vi "print.vi"(6 "ShowType?":bool, 8 "error in (no error)":errorcluster, 11 "Expression":T1) -> (0 "error out":errorcluster, 3 "String":string)   [LabVIEW 2020]
uses:
  ExpressionType.ctl
  Expression.ctl
  ClosureData.ctl
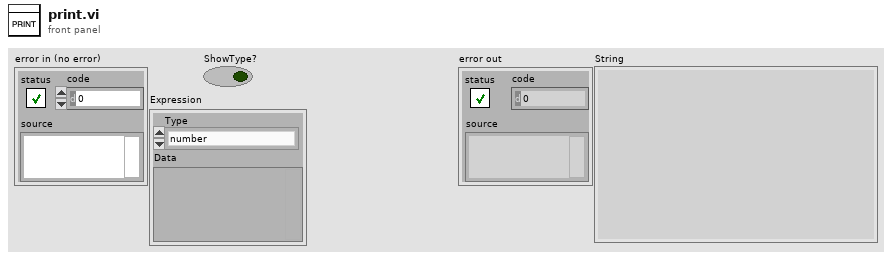
[diagram p1: front panel]
types:
  T1 = typedef "Expression.ctl" = cluster{"Type":T2, "Data":variant}
  T2 = typedef "ExpressionType.ctl" = enum16{"number", "string", "symbol", "primitive", "list", "closure", "macro", "nil", "error"}
  T3 = typedef "ClosureData.ctl" = cluster{"arguments":string[], "code":T1}
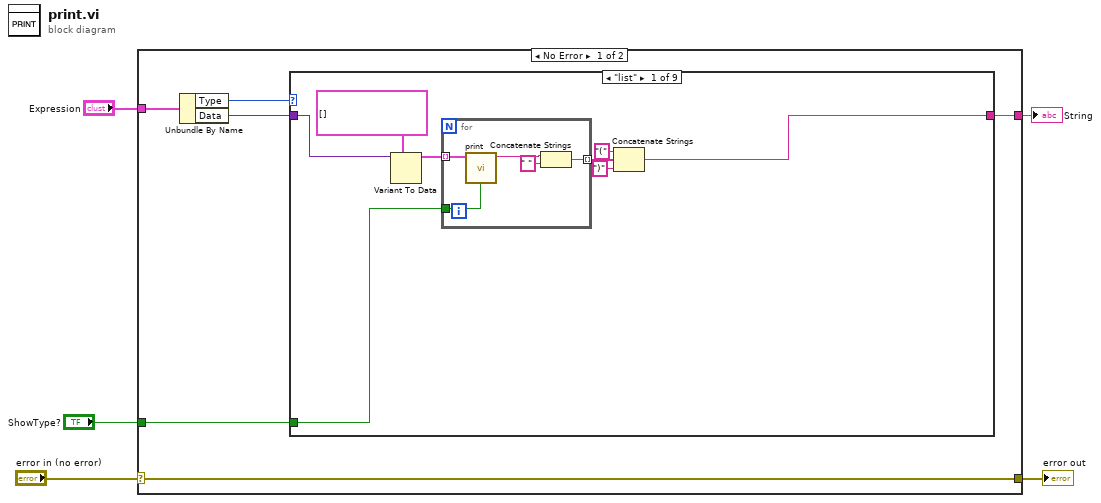
[diagram p0: block diagram]
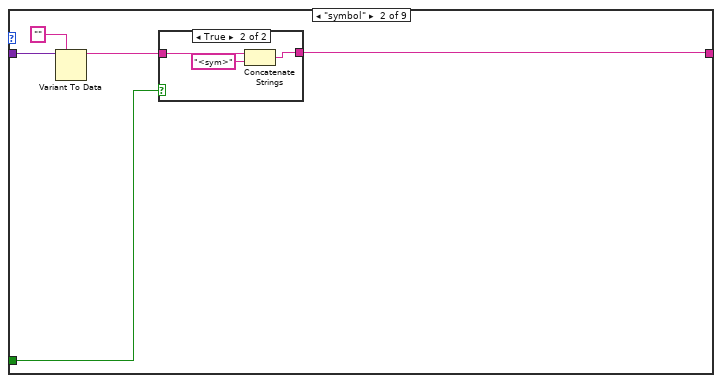
[diagram p2: hidden frame]
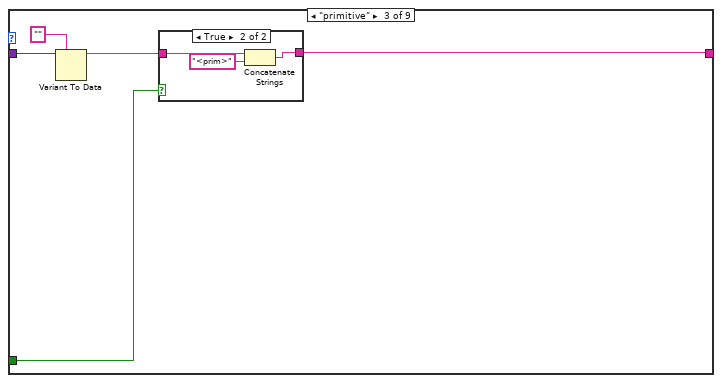
[diagram p4: hidden frame]
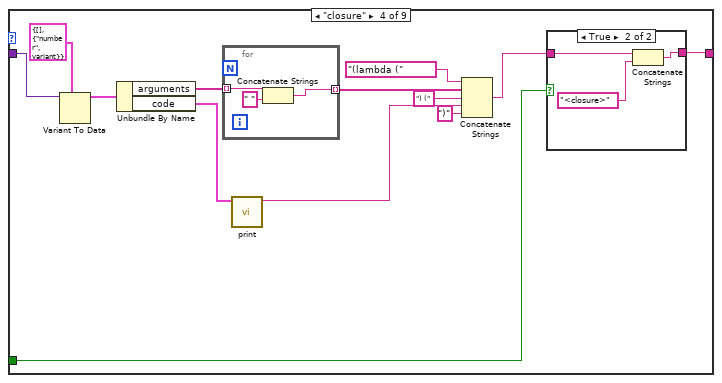
[diagram p6: hidden frame]
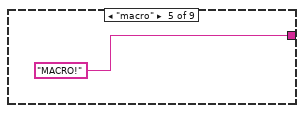
[diagram p8: hidden frame]
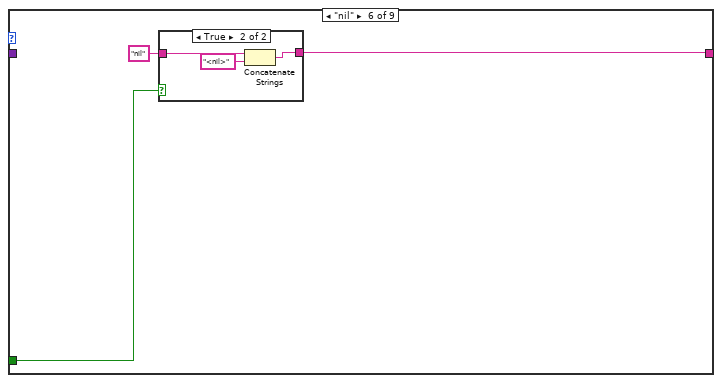
[diagram p9: hidden frame]
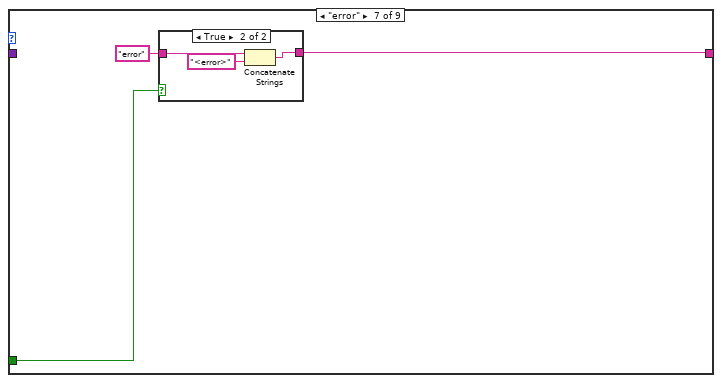
[diagram p11: hidden frame]
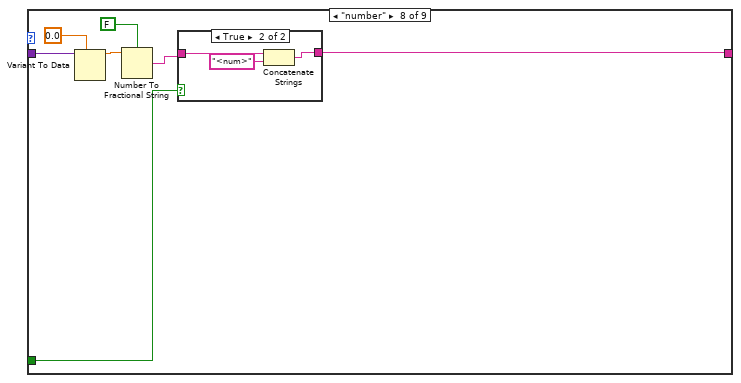
[diagram p13: hidden frame]
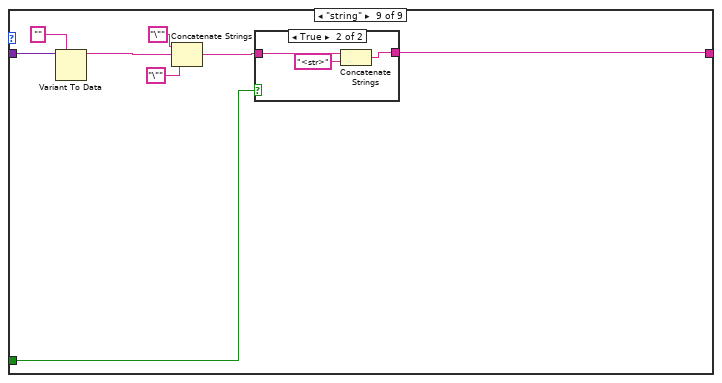
[diagram p15: hidden frame]
diagram:
  n1 = case shown="No Error" "error in (no error)" {
    selector: "error in (no error)" -> [w11 w101]
    tunnel: [w11 w101] -> w4
    tunnel: "Expression" -> [w10 _]
    tunnel: [w7 _] -> w3
    tunnel: "ShowType?" -> [w6 _]
    frame No Error {
      n2 = Unbundle By Name(w10) -> ("Type"=w9:T2, "Data"=w8:variant)
      n3 = case shown="\"list\"" w9 {
        tunnel: w8 -> [w19 w29 w38 w55 _ _ _ w84 w96]
        tunnel: [w14 w26 w35 w54 "MACRO!" w66 w73 w83 w93] -> w7
        tunnel: w6 -> [w13 w25 w34 w53 _ w65 w72 w82 w94]
        frame "list" {
          n4 = Variant To Data(type=T1[] [], Variant=w19) -> (data=w18:T1[])  [unwired: 1 in, 1 out]
          n5 = for {
            tunnel: w18 -> [w22] mode=indexing
            tunnel: [w23] -> w17 mode=indexing
            tunnel: w13 -> [w21]
            n6 = call "print.vi"("ShowType?"=w21, "Expression"=w22) -> ("String"=w20:string)  [unwired: 8 in, 1 out]
            n7 = Concatenate Strings(w20, " " ("string")) -> (w23:string)
          }
          n8 = Concatenate Strings("(" ("string"), w17, ")" ("string")) -> (w14:string)
        }
        frame "symbol" {
          n9 = Variant To Data(type="", Variant=w29) -> (data=w27:string)  [unwired: 1 in, 1 out]
          n10 = case shown="True" w25 {
            tunnel: [w30 w32] -> w26
            tunnel: w27 -> [w30 w33]
            frame False {
            }
            frame True {
              n11 = Concatenate Strings(w33, "<sym>" ("string")) -> (w32:string)
            }
          }
        }
        frame "primitive" {
          n12 = Variant To Data(type="", Variant=w38) -> (data=w36:string)  [unwired: 1 in, 1 out]
          n13 = case shown="True" w34 {
            tunnel: [w39 w41] -> w35
            tunnel: w36 -> [w39 w42]
            frame False {
            }
            frame True {
              n14 = Concatenate Strings(w42, "<prim>" ("string")) -> (w41:string)
            }
          }
        }
        frame "closure" {
          n15 = Variant To Data(type=T3 {"arguments"=[], "code"={"Type"=enum."number", "Data"=variant}} ("ClosureData"), Variant=w55) -> (data=w51:T3)  [unwired: 1 in, 1 out]
          n16 = Unbundle By Name(w51) -> ("arguments"=w49:string[], "code"=w50:T1)
          n17 = for {
            tunnel: w49 -> [w57] mode=indexing
            tunnel: [w56] -> w46 mode=indexing
            n18 = Concatenate Strings(w57, " " ("string")) -> (w56:string)
          }
          n19 = call "print.vi"("Expression"=w50) -> ("String"=w45:string)  [unwired: 9 in, 1 out]
          n20 = Concatenate Strings("(lambda (" ("string"), w46, ") (" ("string"), w45, ")" ("string")) -> (w43:string)
          n21 = case shown="True" w53 {
            tunnel: [w59 w62] -> w54
            tunnel: w43 -> [w59 w60]
            frame False {
            }
            frame True {
              n22 = Concatenate Strings(w60, "<closure>" ("string")) -> (w62:string)
            }
          }
        }
        frame "macro" {
        }
        frame "nil" {
          n23 = case shown="True" w65 {
            tunnel: [w67 w69] -> w66
            tunnel: "nil" -> [w67 w70]
            frame False {
            }
            frame True {
              n24 = Concatenate Strings(w70, "<nil>" ("string")) -> (w69:string)
            }
          }
        }
        frame "error" {
          n25 = case shown="True" w72 {
            tunnel: [w74 w76] -> w73
            tunnel: "error" -> [w74 w77]
            frame False {
            }
            frame True {
              n26 = Concatenate Strings(w77, "<error>" ("string")) -> (w76:string)
            }
          }
        }
        frame "number" {
          n27 = Variant To Data(type=0.0, Variant=w84) -> (data=w80:dbl)  [unwired: 1 in, 1 out]
          n28 = Number To Fractional String(use system decimal point (T)=FALSE, number=w80) -> (F-format string=w79:string)  [unwired: 2 in]
          n29 = case shown="True" w82 {
            tunnel: [w85 w87] -> w83
            tunnel: w79 -> [w85 w88]
            frame False {
            }
            frame True {
              n30 = Concatenate Strings(w88, "<num>" ("string")) -> (w87:string)
            }
          }
        }
        frame "string" {
          n31 = Variant To Data(type="", Variant=w96) -> (data=w90:string)  [unwired: 1 in, 1 out]
          n32 = Concatenate Strings("\"" ("string"), w90, "\"" ("string")) -> (w89:string)
          n33 = case shown="True" w94 {
            tunnel: [w97 w99] -> w93
            tunnel: w89 -> [w97 w100]
            frame False {
            }
            frame True {
              n34 = Concatenate Strings(w100, "<str>" ("string")) -> (w99:string)
            }
          }
        }
      }
    }
    frame Error {
      # "Wire the error cluster across even in the \"No Error\"\ncase so that warnings get propagated."
    }
  }
  "error out" <- w4
  "String" <- w3
